vi "Sample 1 - Basics.vi"() -> ()   [LabVIEW 2016]
panel:
  out "DLL Version":string
  out "System Index":u32
  in  "System Locator":string="usb:ix:0"
  out "Error":errorcluster
  out "Sensor Power-Mode":T1(ring)
  # "Set a system locator here for addressing the MCS.\nA USB MCS locator has the form \"usb:id:123456789\" or \"usb:ix:0\",\na network MCS locator is written \"network:192.168.1.200:5000\"."
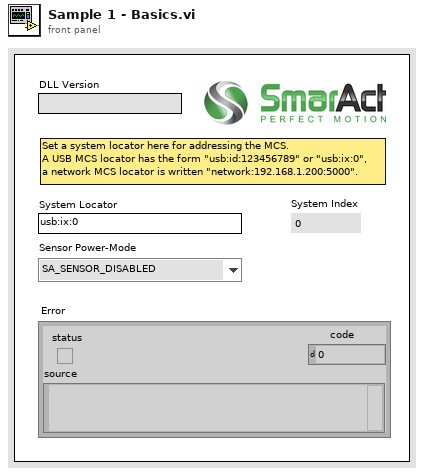
[diagram p1: front panel]
types:
  T1 = enum32{"SA_SENSOR_DISABLED", "SA_SENSOR_ENABLED", "SA_SENSOR_POWERSAVE"}
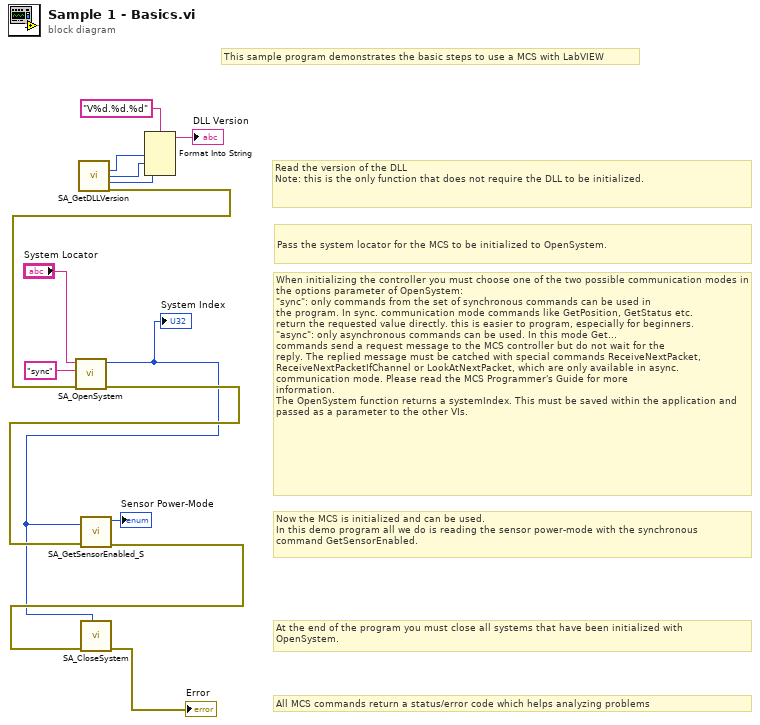
[diagram p0: block diagram]
diagram:
  # "Read the version of the DLL\nNote: this is the only function that does not require the DLL to be initialized."
  # "All MCS commands return a status/error code which helps analyzing problems"
  # "At the end of the program you must close all systems that have been initialized with \nOpenSystem."
  # "Now the MCS is initialized and can be used.\nIn this demo program all we do is reading the sensor power-mode with the synchronous\ncommand GetSensorEnabled."
  # "Pass the system locator for the MCS to be initialized to OpenSystem."
  # "This sample program demonstrates the basic steps to use a MCS with LabVIEW"
  # "When initializing the controller you must choose one of the two possible communication modes in the options parameter of OpenSystem:\n\"sync\": only commands from the set of synchronous commands can be used in\nthe program. In sync. communication mode commands like GetPosition, GetStatus etc.\nreturn the requested value directly. this is easier to program, especially for beginners.\n\"async\": only asynchronous commands can be used. In this mode Get... \ncommands send a request message to the MCS controller but do not wait for the\nreply. The replied message must be catched with special commands ReceiveNextPacket,\nReceiveNextPacketIfChannel or LookAtNextPacket, which are only available in async.\ncommunication mode. Please read the MCS Programmer's Guide for more\ninformation.\nThe OpenSystem function returns a systemIndex. This must be saved within the application and passed as a parameter to the other VIs."
  n1 = call <vilib>:"SA_GetDLLVersion.vi"() -> ("hiVersion"=w3:u32, "loVersion"=w2:u32, "buildVersion"=w1:u32, "error out"=w6:errorcluster)  [unwired: 11 in, 1 out]
  n2 = call <vilib>:"SA_OpenSystem.vi"("error in (no error)"=w6, "options"="sync", "systemLocator"="System Locator") -> ("error out"=w10:errorcluster, "systemIndexOut"=w7:u32)  [unwired: 7 in]
  "System Index" <- w7
  n3 = call <vilib>:"SA_GetSensorEnabled_S.vi"("systemIndex"=w7, "error in (no error)"=w10) -> ("error out"=w9:errorcluster, "enabled"=→"Sensor Power-Mode":T1)  [unwired: 8 in]
  n4 = call <vilib>:"SA_CloseSystem.vi"("systemIndex"=w7, "error in (no error)"=w9) -> ("error out"=→"Error":errorcluster)  [unwired: 9 in]
  n5 = Format Into String(format string="V%d.%d.%d", w3, w2, w1) -> (resulting string=→"DLL Version":string)  [unwired: 2 in, 1 out]
